vi "OnDeviceSelectedyes.vi"(8 "error in":errorcluster, 9 "Device Array":T2(array[cluster]), 10 "UI":T1, 11 "CmdLib In":refnum<k24>) -> (0 "error out":errorcluster)   [LabVIEW 2021]
uses:
  C:/Program Files/New Focus/New Focus Picomotor Application/Samples/LabVIEW/Model 8742/LabVIEW 2009/CmdLib.dll
  Global Variablesyes.vi
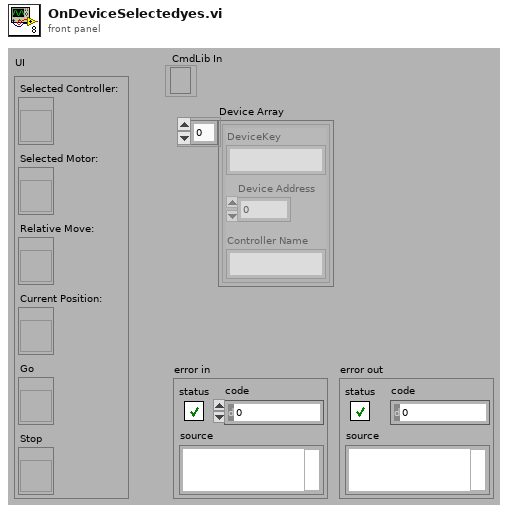
[diagram p1: front panel]
types:
  T1 = cluster{"Selected Controller:":refnum<vi>, "Selected Motor:":refnum<vi>, "Relative Move:":refnum<vi>, "Current Position:":refnum<vi>, "Go":refnum<vi>, "Stop":refnum<vi>}
  T2 = cluster{"DeviceKey":string, "Device Address":i32, "Controller Name":string}[]
  T3 = cluster{"DeviceKey":string, "Device Address":i32, "Controller Name":string}
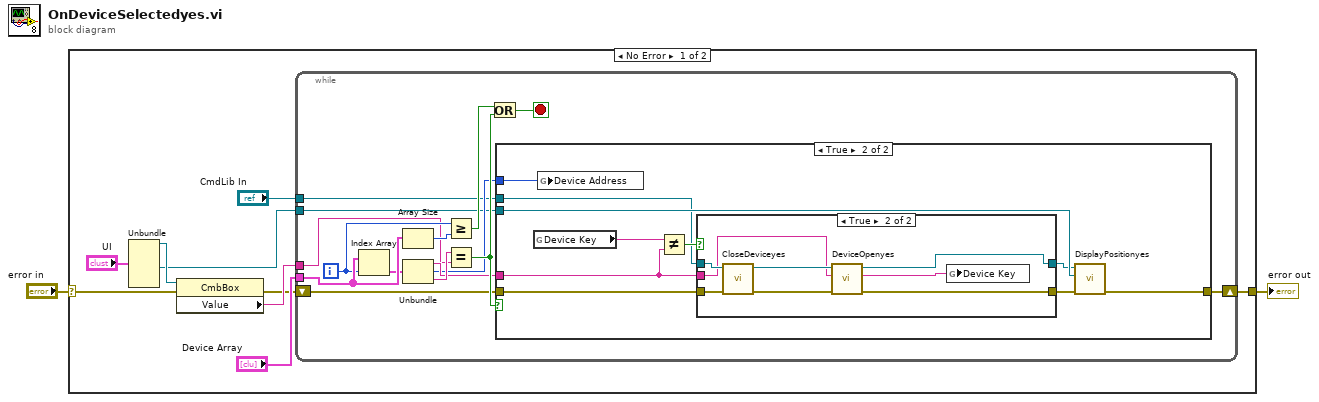
[diagram p0: block diagram]
diagram:
  n1 = case shown="No Error" "error in" {
    selector: "error in" -> [w8 w48]
    tunnel: [w10 w48] -> w2
    frame No Error {
      n2 = Unbundle("UI") -> ("Selected Controller:"=w5:refnum<vi>, "Current Position:"=w4:refnum<vi>)  [unwired: 4 out]
      n3 = property class="CmbBox"(reference=w5, error in=w8) -> (error out=w6:errorcluster, "Value"=w9:string)  [unwired: 1 out]
      n4 = while {
        tunnel: "Device Array" -> [w25]
        tunnel: w9 -> [w12]
        tunnel: w4 -> [w14]
        shift-right: [w16] -> w10
        shift-left: w6 -> [w15]
        tunnel: "CmdLib In" -> [w13]
        i -> [w24]
        stop <- w19 stop-if-true
        n5 = Index Array(array=w25, index=w24) -> (element=w23:T3)
        n6 = Array Size(array=w25) -> (size(s)=w26:i32)
        n7 = Unbundle(w23) -> ("DeviceKey"=w18:string, "Device Address"=w17:i32, "Controller Name"=w22:string)
        n8 = Greater Or Equal?(x=w24, y=w26) -> (x >= y?=w21:bool)
        n9 = Equal?(x=w22, y=w12) -> (x = y?=w20:bool)
        n10 = Or(x=w21, y=w20) -> (x .or. y?=w19:bool)
        n11 = case shown="True" w20 {
          tunnel: w18 -> [_ w33]
          tunnel: w17 -> [_ w30]
          tunnel: [w27 w37] -> w16
          tunnel: w15 -> [w27 w35]
          tunnel: w14 -> [_ w36]
          tunnel: w13 -> [_ w31]
          frame False {
          }
          frame True {
            n12 = global read "Global Variablesyes.vi" "Device Key"() -> (w34:string)
            n13 = global write "Global Variablesyes.vi" "Device Address"(w30) -> ()
            n14 = Not Equal?(x=w34, y=w33) -> (x != y?=w32:bool)
            n15 = case shown="True" w32 {
              tunnel: [w39 w41] -> w28
              tunnel: w31 -> [w38 w47]
              tunnel: w35 -> [w39 w45]
              tunnel: w33 -> [_ w43]
              tunnel: [w38 w40] -> w29
              frame False {
              }
              frame True {
                n16 = call "CloseDeviceyes.vi"("error in"=w45, "CmdLib In"=w47) -> ("error out"=w46:errorcluster, "CmdLib Out"=w44:refnum<k24>)  [unwired: 8 in]
                n17 = call "DeviceOpenyes.vi"("error in (no error)"=w46, "DeviceKey In"=w43, "CmdLib In"=w44) -> ("error out"=w41:errorcluster, "DeviceKey Out"=w42:string, "CmdLib Out"=w40:refnum<k24>)  [unwired: 2 in]
                n18 = global write "Global Variablesyes.vi" "Device Key"(w42) -> ()
              }
            }
            n19 = call "DisplayPositionyes.vi"("error in"=w28, "Current Position:"=w36, "CmdLib In"=w29) -> ("error out"=w37:errorcluster)  [unwired: 7 in, 1 out]
          }
        }
      }
    }
    frame Error {
    }
  }
  "error out" <- w2
